vi "Add Target to Items Map.vi"(8 "error in (no error)":errorcluster, 9 "Order":i32, 11 "ProjectItem Ref":refnum<vi>) -> (0 "error out":errorcluster, 2 "Descendents Refs":refnum<vi>[](array[refnum]), 3 "Item":refnum<class "Item.lvclass">)   [LabVIEW 2020, in "VI Properties Editor.lvlib"]
uses:
  Classes/Item/Item.lvclass
  VI Properties Editor.lvlib
  Classes/Support/Item Type.ctl
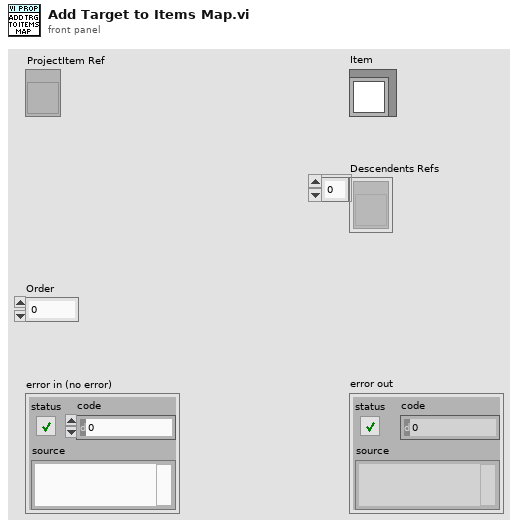
[diagram p1: front panel]
types:
  T1 = typedef "VI Properties Editor.lvlib/Item Type.ctl" = enum16{"Generic", "VI"}
  T2 = typedef "imagedata.ctl" = cluster{"image type":i32, "image depth":i32, "image":u8[], "mask":u8[], "colors":u32[], "Rectangle":cluster{"left":i16, "top":i16, "right":i16, "bottom":i16}}
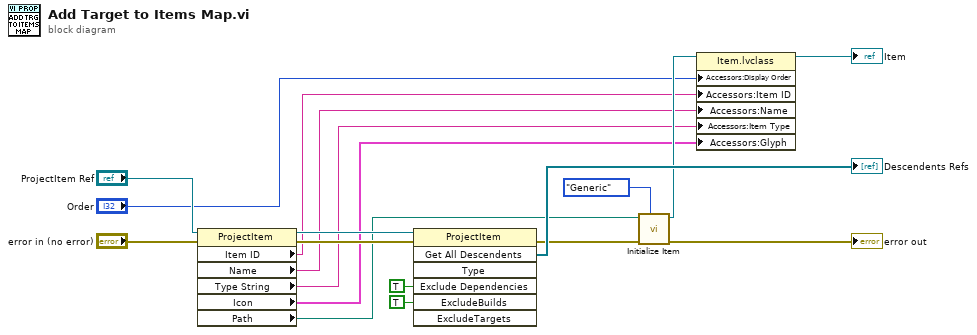
[diagram p0: block diagram]
diagram:
  n1 = property class="ProjectItem"(reference="ProjectItem Ref", error in="error in (no error)") -> (reference out=w14:refnum<vi>, error out=w18:errorcluster, "Item ID"=w7:string, "Name"=w6:string, "Type String"=w5:string, "Icon"=w4:T2, "Path"=w3:path)
  n2 = invoke class="ProjectItem" method="Get All Descendents"(reference=w14, error in=w18, "Exclude Dependencies"=TRUE ("ExcludeDependencies"), "ExcludeBuilds"=TRUE) -> (error out=w10:errorcluster, "All Descendents"=→"Descendents Refs":refnum<vi>[])  [unwired: 3 in, 5 out]
  n3 = call "Initialize Item.vi"("Item Type"=Item_Type."Generic", "error in (no error)"=w10, "Path"=w3) -> ("error out"=→"error out":errorcluster, "Item"=w9:refnum<class "Item.lvclass">)  [unwired: 7 in]
  n4 = property class="Item.lvclass"(reference=w9, "Accessors:Display Order"="Order", "Accessors:Item ID"=w7, "Accessors:Name"=w6, "Accessors:Item Type"=w5, "Accessors:Glyph"=w4) -> (reference out=→"Item":refnum<class "Item.lvclass">)  [unwired: 1 in, 1 out]
